vi "Add Instrument.vi"(8 "error in":errorcluster, 10 "Instrument":refnum<class "Instrument.lvclass">, 11 "MSS in":refnum<class "MSS.lvclass">) -> (0 "error out":errorcluster, 3 "MSS out":refnum<class "MSS.lvclass">)   [LabVIEW 2024, in "HAL.lvlib" / "MSS.lvclass"]
uses:
  MSS.lvclass
  Instrument/Instrument.lvclass
  MSS.lvclass/MSS.ctl
  <vilib>/Utility/miscctls.llb/LVMapReplaceAction.ctl
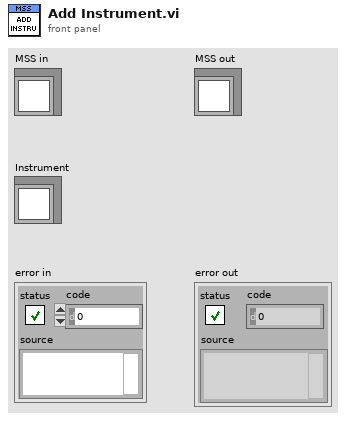
[diagram p1: front panel]
types:
  T1 = typedef "LVMapReplaceAction.ctl" = enum32{"Modify Entry only if found", "Add or Modify Entry", "Delete Entry"}
  T2 = map{string, cluster{"Instrument":refnum<class "Instrument.lvclass">, "Ref Count":i16}}
  T3 = cluster{"Instrument":refnum<class "Instrument.lvclass">, "Ref Count":i16}
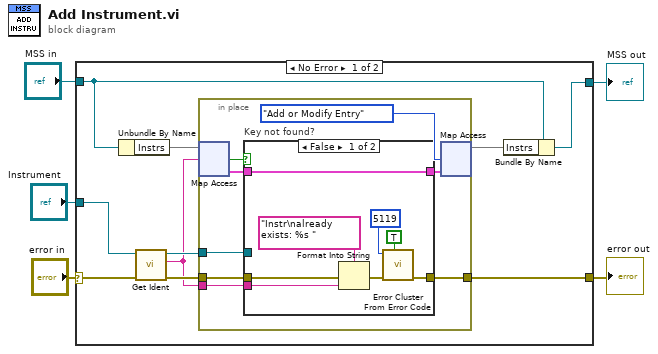
[diagram p0: block diagram]
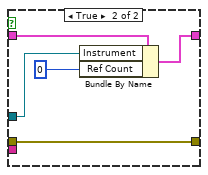
[diagram p2: hidden frame]
diagram:
  n1 = case shown="No Error" "error in" {
    selector: "error in" -> [w7 w38]
    tunnel: "Instrument" -> [w15 _]
    tunnel: "MSS in" -> [w10 w37]
    tunnel: [w9 w37] -> w4
    tunnel: [w8 w38] -> w3
    frame No Error {
      n2 = Unbundle By Name(w10) -> ("Instrs"=w13:T2)
      n3 = call "Get Ident.vi"("Error In"=w7, "reference in"=w15) -> ("Error Out"=w11:errorcluster, "Ident"=w6:string, "reference out"=w12:refnum<class "Instrument.lvclass">)  [unwired: 7 in]
      n4 = in-place {
        in-place-border: w12 -> [w21]
        in-place-border: w11 -> [w18]
        in-place-border: [w17] -> w8
        in-place-border: w6 -> [w16]
        n5 = in-place-map #1(w13, w6) -> (w22:T3, w23:bool)  [unwired: 1 in]
        n6 = case "Key not found?" shown="False" w23 {
          tunnel: w22 -> [w30 w33]
          tunnel: [w30 w35] -> w19
          tunnel: w21 -> [_ w36]
          tunnel: w18 -> [w31 w34]
          tunnel: [w29 w34] -> w17
          tunnel: w16 -> [w25 _]
          frame False {
            n7 = Format Into String(format string="Instr\nalready exists: %s ", error in=w31, w25) -> (error out=w27:errorcluster)  [unwired: 1 in, 1 out]
            n8 = call <vilib>:"Error Cluster From Error Code.vi"("show call chain? (False)"=TRUE, "error in (no error)"=w27, "error code (0)"=5119) -> ("error out"=w29:errorcluster)  [unwired: 6 in]
          }
          frame True {
            n9 = Bundle By Name(cluster=w33, "Instrument"=w36, "Ref Count"=u8 0) -> (w35:T3)
          }
        }
        n10 = in-place-map #1(w19, LVMapReplaceAction."Add or Modify Entry" ("action")) -> (w14:T2)  [unwired: 2 out]
      }
      n11 = Bundle By Name(cluster=w10, "Instrs"=w14) -> (w9:refnum<class "MSS.lvclass">)
    }
    frame Error {
    }
  }
  "error out" <- w3
  "MSS out" <- w4
